vi "Format Argument Error.vi"(7 "Error Type":T1(ring), 9 "Value":string, 10 "Name":string) -> (2 "String":string)   [LabVIEW 2020, in "LV ArgParse.lvlib" / "LV Argument Parser.lvclass"]
uses:
  LV Argument Parser.lvclass
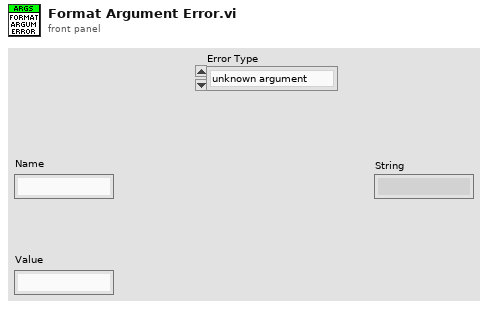
[diagram p1: front panel]
types:
  T1 = enum16{"unknown argument", "invalid argument type", "wrong argument count", "missing required argument"}
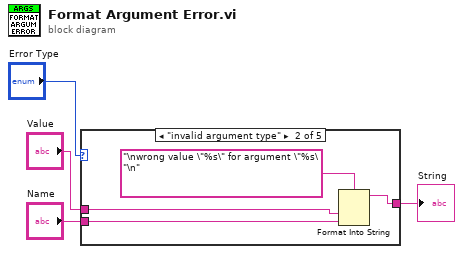
[diagram p0: block diagram]
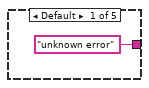
[diagram p2: hidden frame]
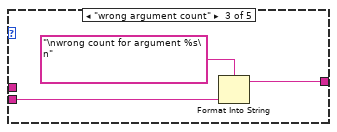
[diagram p3: hidden frame]
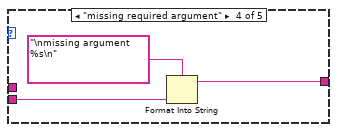
[diagram p4: hidden frame]
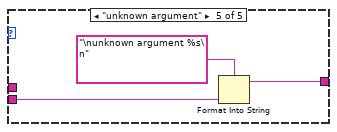
[diagram p5: hidden frame]
diagram:
  n1 = case shown="\"invalid argument type\"" "Error Type" {
    tunnel: "Name" -> [_ w8 w10 w13 w16]
    tunnel: "Value" -> [_ w7 _ _ _]
    tunnel: ["unknown error" w6 w11 w14 w17] -> w1
    frame Default {
    }
    frame "invalid argument type" {
      n2 = Format Into String(format string="\nwrong value \"%s\" for argument \"%s\"\n", w7, w8) -> (resulting string=w6:string)  [unwired: 2 in, 1 out]
    }
    frame "wrong argument count" {
      n3 = Format Into String(format string="\nwrong count for argument %s\n", w10) -> (resulting string=w11:string)  [unwired: 2 in, 1 out]
    }
    frame "missing required argument" {
      n4 = Format Into String(format string="\nmissing argument %s\n", w13) -> (resulting string=w14:string)  [unwired: 2 in, 1 out]
    }
    frame "unknown argument" {
      n5 = Format Into String(format string="\nunknown argument %s\n", w16) -> (resulting string=w17:string)  [unwired: 2 in, 1 out]
    }
  }
  "String" <- w1
